vi "ezAFM Practice 1.4.vi"() -> ()   [LabVIEW 2015]
uses:
  D:/LabVIEW for ezAFM/LV-PGC 2019-05a/Special Equipment/ezAFM/NMI Integration Code/ezCommander.dll
  LabVIEW for ezAFM/LV-PGC 2019-05a/Special Equipment/ezAFM/NMI Integration Code/ezCommander.dll
  <vilib>/userdefined/High Color/IMAQdx.ctl
  LabVIEW for ezAFM/LV-PGC 2019-05a/Universal vi's/Global Variables/Globals-EasyAFM.vi
  Globals.vi
  <vilib>/vision/driver/NI_Vision_Acquisition_Software.lvlib
panel:
  in  "Camera":enum32{"ezAFM Camera"}(tab)
  out "ezAFM Camera":T1(plugin-control)
  out "XY Vector":dbl[](array[numeric])
  in  "Main Menu":enum32{"Navigation", "Scanning"}(tab)
  in  "APPROACH":bool
  in  "RETRACT":bool
  in  "Step Size":dbl
  out "Angle":dbl
  in  "THETA":bool
  in  "MOVE":bool
  in  "Current Device":string(combo)
  in  "Target Device":string(combo)
  in  "Motor Speed":u16(ring)=5000 items=["SLOW"=5000, "MEDIUM"=30000, "FAST"=50000]
  in  "Navigation Buttons":T2
  in  "QUIT":bool
  in  "UPDATE DEVICE":bool
  out "Scan Spot":string
  in  "Leads":string(combo)
  in  "Device":string(combo)
  in  "Chip":string
  in  "Image Resolution":u16(ring)=256 items=["32"=32, "64"=64, "128"=128, "256"=256, "512"=512, "1024"=1024, "2048"=2048]
  in  "SELECT CONNECTIONS":bool
  in  "BEGIN SCAN":bool
  out "Current Device to Scan":string
  out "Connections":string[](array[string])
  in  "Indicators":enum32{"Indicators"}(tab)
  out "XYZ Motor Position":dbl[](array[numeric])
  out "ezAFM Status":dbl
  out "Approaching":bool
  out "ezAFM Connected":bool
  out "Retracting":bool
  out "Scanning":bool
  out "Tip Approached?":bool
  in  "RESET":bool
  out "XY Position":dbl[](array[numeric])
  # "Use Arrow Keys to manually\nmove the XY Motor"
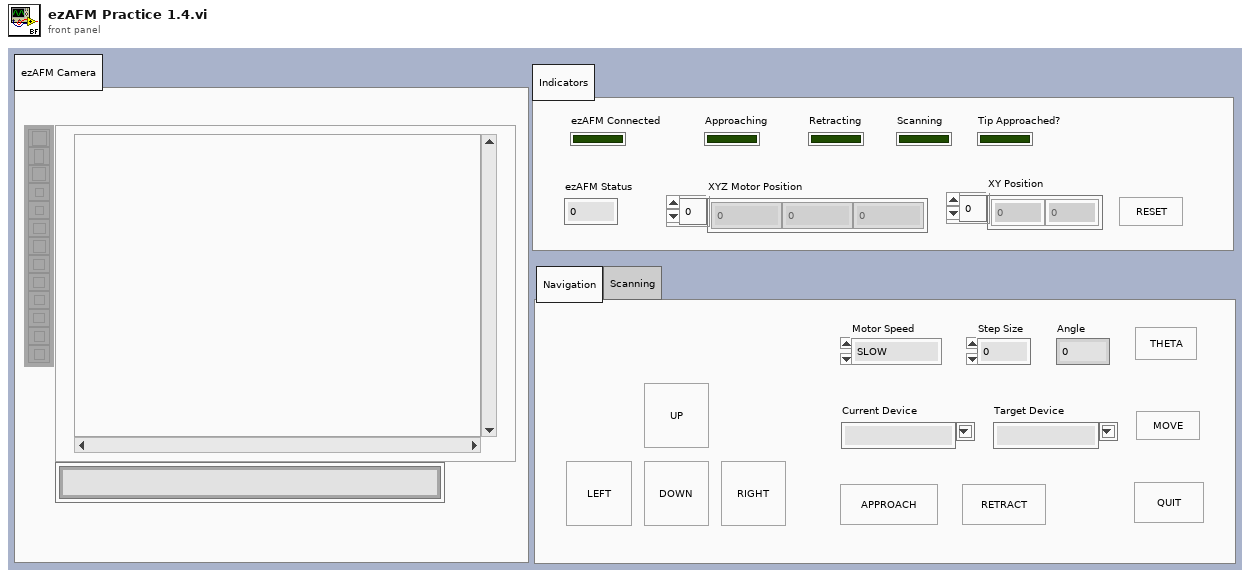
[diagram p1: front panel]
types:
  T1 = typedef "IMAQ Image.ctl" = refnum<image>
  T2 = cluster{"UP":bool, "DOWN":bool, "LEFT":bool, "RIGHT":bool}
  T3 = typedef "IMAQdx.ctl" = refnum<k21>
  T4 = typedef "Image Type" = u32
  T5 = typedef "eventvkey.ctl" = enum16{"ASCII", "Enter", "Return", "Shift", "Ctrl", "Alt", "Cmd", "Opt", "Caps", "NumLock", "Clear", "Break", "Up", "Down", "Left", "Right", "Insert", "Delete", "Home", "End", "PageUp", "PageDown", "Escape", "Help", "Pause", "ScrollLock", "F1", "F2", "F3", "F4", "F5", "F6", "F7", "F8", "F9", "F10", "F11", "F12", "F13", "F14", "F15", "F16", "F17", "F18", "F19", "F20", "F21", "F22", "F23", "F24", "Play", "VolumeUp", "VolumeDown", "Mute", "Two Byte Char"}
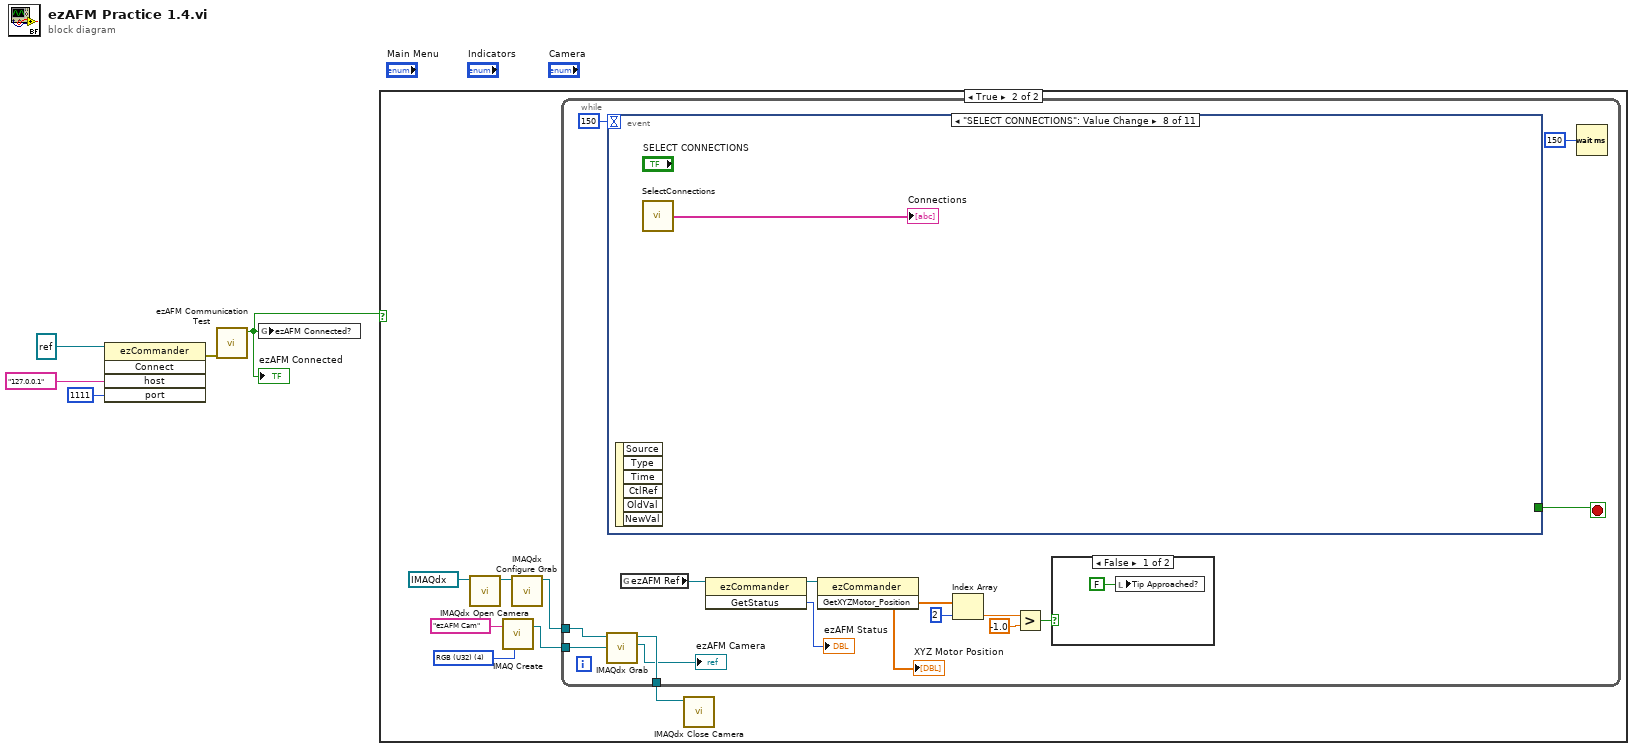
[diagram p0: block diagram]
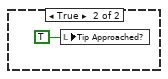
[diagram p3: hidden frame]
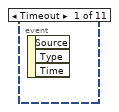
[diagram p4: hidden frame]
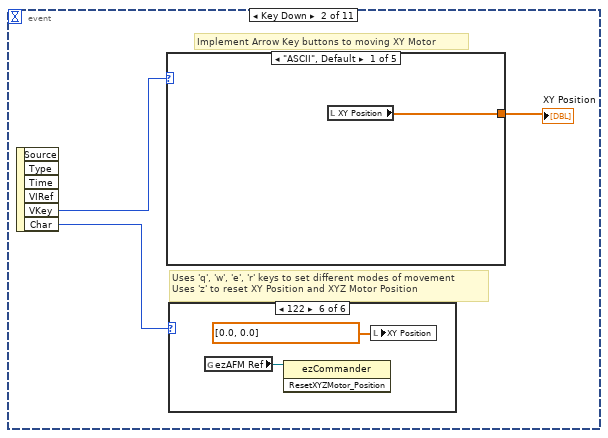
[diagram p5: hidden frame]
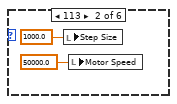
[diagram p7: hidden frame]
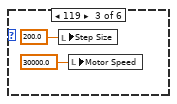
[diagram p8: hidden frame]
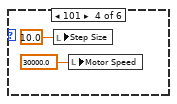
[diagram p9: hidden frame]
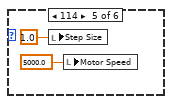
[diagram p10: hidden frame]
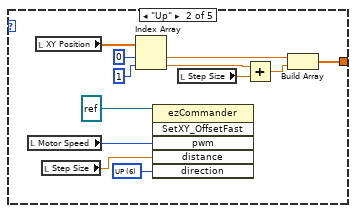
[diagram p11: hidden frame]
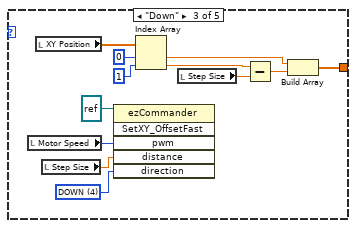
[diagram p12: hidden frame]
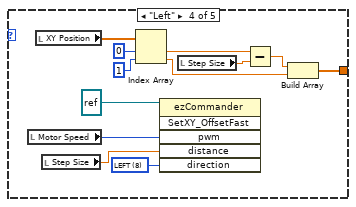
[diagram p13: hidden frame]
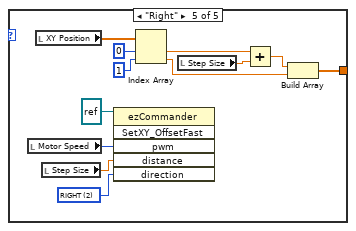
[diagram p14: hidden frame]
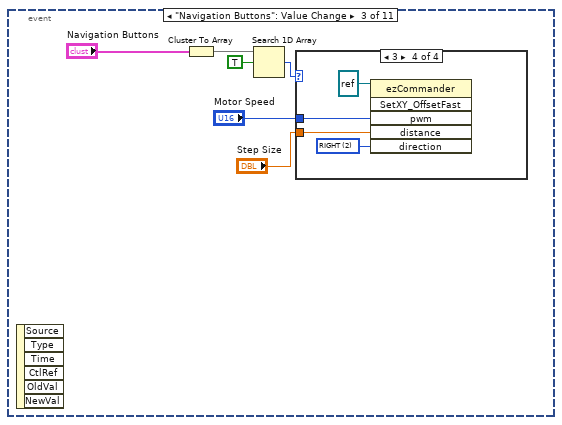
[diagram p15: hidden frame]
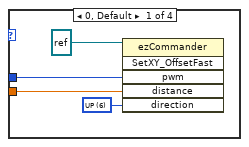
[diagram p16: hidden frame]
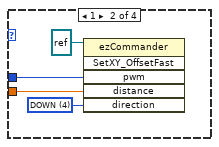
[diagram p17: hidden frame]
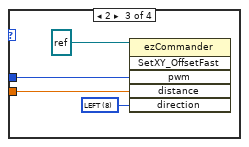
[diagram p18: hidden frame]
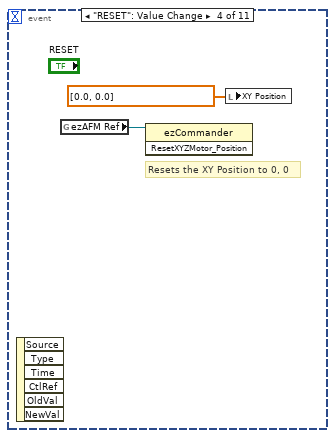
[diagram p19: hidden frame]
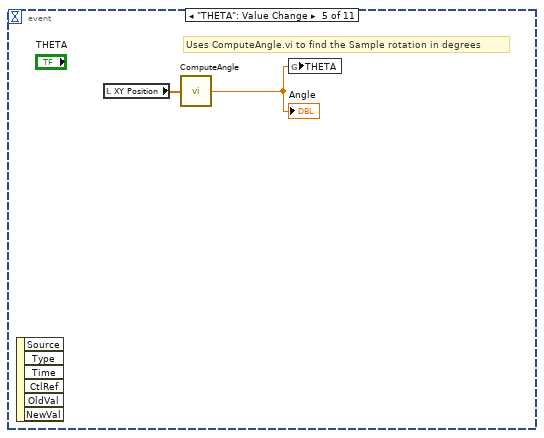
[diagram p20: hidden frame]
diagram:
  n1 = invoke class="ezCommander" method="Connect"(reference=refnum<k24> refnum ("ezAFM Ref"), "host"="127.0.0.1", "port"=1111) -> (error out=w4:errorcluster)  [unwired: 2 in, 4 out]
  n2 = call "ezAFM Communication Test.vi"("error in"=w4) -> ("ezAFM COM status"=w1:bool)  [unwired: 3 in, 3 out]
  "ezAFM Connected" <- w1
  n3 = global write "Globals.vi" "ezAFM Connected?"(w1) -> ()
  n4 = case shown="True" w1 {
    frame False {
    }
    frame True {
      w6 = T4 4 items=["Grayscale (U8)", "Grayscale (I16)", "Grayscale (SGL)", "Complex (CSG)", "RGB (U32)", "HSL (U32)", "RGB (U64)", "Grayscale (U16)"] ("Image Type")
      n5 = call <vilib>:"IMAQdx Open Camera.vi"("Session In"=T3 "cam5") -> ("Session Out"=w10:T3)  [unwired: 9 in, 1 out]
      n6 = call "IMAQ Create"("Image Name"="ezAFM Cam", "Image Type"=w6) -> ("New Image"=w9:T1)  [unwired: 3 in, 1 out]
      n7 = call <vilib>:"IMAQdx Configure Grab.vi"("Session In"=w10) -> ("Session Out"=w8:T3)  [unwired: 9 in, 1 out]
      n8 = while {
        tunnel: w9 -> [w17]
        tunnel: w8 -> [w16]
        tunnel: [w15] -> w7
        stop <- w20 stop-if-true
        n9 = call <vilib>:"IMAQdx Grab.vi"("Image In"=w17, "Session In"=w16) -> ("Image Out"=→"ezAFM Camera":T1, "Session Out"=w15:T3)  [unwired: 2 in, 6 out]
        n10 = event shown="[7] \"SELECT CONNECTIONS\": Value Change" {
          selector: _ -> [_ _ _ _ _ _ _ _ _ _ _]
          dyn-events: _ -> [_ _ _ _ _ _ _ _ _ _ _]
          timeout: 150 -> [_ _ _ _ _ _ _ _ _ _ _]
          tunnel: [_ _ _ _ _ _ _ _ _ _ "QUIT"] -> w20
          event Timeout {
            n11 = event-data() -> ()  [unwired: 1 in, 3 out]
          }
          event Key Down {
            # "Uses 'q', 'w', 'e', 'r' keys to set different modes of movement\nUses 'z' to reset XY Position and XYZ Motor Position"
            # "Implement Arrow Key buttons to moving XY Motor"
            n12 = event-data() -> ("VKey"=w30:T5, "Char"=w31:i16)  [unwired: 1 in, 4 out]
            n13 = case shown="\"ASCII\", Default" w30 {
              tunnel: [w43 w44 w56 w68 w80] -> w32
              frame "ASCII", Default {
                n14 = local read "XY Position"() -> (w43:dbl[])
              }
              frame "Up" {
                w54 = u16 6 items=["UP"=6, "DOWN"=4, "LEFT"=8, "RIGHT"=2]
                n15 = local read "Motor Speed"() -> (w53:u16)
                n16 = local read "XY Position"() -> (w51:dbl[])
                n17 = local read "Step Size"() -> (w52:dbl)
                n18 = Index Array(array=w51, index #1=0 ("index"), index #2=1 ("index")) -> (element #1=w46:dbl, element #2=w47:dbl)
                n19 = invoke class="ezCommander" method="SetXY_OffsetFast"(reference=refnum<k24> refnum ("ezAFM Ref"), "pwm"=w53, "distance"=w52, "direction"=w54) -> ()  [unwired: 2 in, 6 out]
                n20 = local read "Step Size"() -> (w48:dbl)
                n21 = Add(x=w47, y=w48) -> (x+y=w45:dbl)
                n22 = Build Array(w46, w45) -> (w44:dbl[])
              }
              frame "Down" {
                w64 = u16 4 items=["UP"=6, "DOWN"=4, "LEFT"=8, "RIGHT"=2]
                n23 = local read "Motor Speed"() -> (w66:u16)
                n24 = local read "XY Position"() -> (w58:dbl[])
                n25 = local read "Step Size"() -> (w65:dbl)
                n26 = invoke class="ezCommander" method="SetXY_OffsetFast"(reference=refnum<k24> refnum ("ezAFM Ref"), "pwm"=w66, "distance"=w65, "direction"=w64) -> ()  [unwired: 2 in, 6 out]
                n27 = Index Array(array=w58, index #1=0 ("index"), index #2=1 ("index")) -> (element #1=w60:dbl, element #2=w61:dbl)
                n28 = local read "Step Size"() -> (w57:dbl)
                n29 = Subtract(x=w61, y=w57) -> (x-y=w59:dbl)
                n30 = Build Array(w60, w59) -> (w56:dbl[])
              }
              frame "Left" {
                w78 = u16 8 items=["UP"=6, "DOWN"=4, "LEFT"=8, "RIGHT"=2]
                n31 = local read "Motor Speed"() -> (w76:u16)
                n32 = local read "XY Position"() -> (w72:dbl[])
                n33 = local read "Step Size"() -> (w77:dbl)
                n34 = Index Array(array=w72, index #1=0 ("index"), index #2=1 ("index")) -> (element #1=w71:dbl, element #2=w69:dbl)
                n35 = invoke class="ezCommander" method="SetXY_OffsetFast"(reference=refnum<k24> refnum ("ezAFM Ref"), "pwm"=w76, "distance"=w77, "direction"=w78) -> ()  [unwired: 2 in, 6 out]
                n36 = local read "Step Size"() -> (w73:dbl)
                n37 = Subtract(x=w71, y=w73) -> (x-y=w70:dbl)
                n38 = Build Array(w70, w69) -> (w68:dbl[])
              }
              frame "Right" {
                w90 = u16 2 items=["UP"=6, "DOWN"=4, "LEFT"=8, "RIGHT"=2]
                n39 = local read "Motor Speed"() -> (w89:u16)
                n40 = local read "XY Position"() -> (w85:dbl[])
                n41 = local read "Step Size"() -> (w88:dbl)
                n42 = invoke class="ezCommander" method="SetXY_OffsetFast"(reference=refnum<k24> refnum ("ezAFM Ref"), "pwm"=w89, "distance"=w88, "direction"=w90) -> ()  [unwired: 2 in, 6 out]
                n43 = Index Array(array=w85, index #1=0 ("index"), index #2=1 ("index")) -> (element #1=w83:dbl, element #2=w81:dbl)
                n44 = local read "Step Size"() -> (w84:dbl)
                n45 = Add(x=w83, y=w84) -> (x+y=w82:dbl)
                n46 = Build Array(w82, w81) -> (w80:dbl[])
              }
            }
            "XY Position" <- w32
            n47 = case shown="122" w31 {
              frame 0, Default {
              }
              frame 113 {
                n48 = local write "Step Size"(1000.0 ("Step Size")) -> ()
                n49 = local write "Motor Speed"(50000.0 ("Motor Speed")) -> ()
              }
              frame 119 {
                n50 = local write "Step Size"(200.0 ("Step Size")) -> ()
                n51 = local write "Motor Speed"(30000.0 ("Motor Speed")) -> ()
              }
              frame 101 {
                n52 = local write "Step Size"(10.0 ("Step Size")) -> ()
                n53 = local write "Motor Speed"(30000.0 ("Motor Speed")) -> ()
              }
              frame 114 {
                n54 = local write "Step Size"(1.0 ("Step Size")) -> ()
                n55 = local write "Motor Speed"(5000.0 ("Motor Speed")) -> ()
              }
              frame 122 {
                n56 = global read "Globals-EasyAFM.vi" "ezAFM Ref"() -> (w41:refnum<k24>)
                n57 = invoke class="ezCommander" method="ResetXYZMotor_Position"(reference=w41) -> ()  [unwired: 2 in, 3 out]
                n58 = local write "XY Position"(dbl[] [0.0, 0.0] ("XY Position")) -> ()
              }
            }
          }
          event "Navigation Buttons": Value Change {
            n59 = event-data() -> ()  [unwired: 1 in, 6 out]
            n60 = Cluster To Array(cluster="Navigation Buttons") -> (array=w96:bool[])
            n61 = Search 1D Array(1D array=w96, element=TRUE) -> (index of element=w94:i32)  [unwired: 1 in]
            n62 = case shown="3" w94 {
              tunnel: "Step Size" -> [w98 w103 w107 w111]
              tunnel: "Motor Speed" -> [w99 w102 w106 w110]
              frame 0, Default {
                w100 = u16 6 items=["UP"=6, "DOWN"=4, "LEFT"=8, "RIGHT"=2]
                n63 = invoke class="ezCommander" method="SetXY_OffsetFast"(reference=refnum<k24> refnum ("ezAFM Ref"), "pwm"=w99, "distance"=w98, "direction"=w100) -> ()  [unwired: 2 in, 6 out]
              }
              frame 1 {
                w104 = u16 4 items=["UP"=6, "DOWN"=4, "LEFT"=8, "RIGHT"=2]
                n64 = invoke class="ezCommander" method="SetXY_OffsetFast"(reference=refnum<k24> refnum ("ezAFM Ref"), "pwm"=w102, "distance"=w103, "direction"=w104) -> ()  [unwired: 2 in, 6 out]
              }
              frame 2 {
                w108 = u16 8 items=["UP"=6, "DOWN"=4, "LEFT"=8, "RIGHT"=2]
                n65 = invoke class="ezCommander" method="SetXY_OffsetFast"(reference=refnum<k24> refnum ("ezAFM Ref"), "pwm"=w106, "distance"=w107, "direction"=w108) -> ()  [unwired: 2 in, 6 out]
              }
              frame 3 {
                w112 = u16 2 items=["UP"=6, "DOWN"=4, "LEFT"=8, "RIGHT"=2]
                n66 = invoke class="ezCommander" method="SetXY_OffsetFast"(reference=refnum<k24> refnum ("ezAFM Ref"), "pwm"=w110, "distance"=w111, "direction"=w112) -> ()  [unwired: 2 in, 6 out]
              }
            }
          }
          event "RESET": Value Change {
            # "Resets the XY Position to 0, 0"
            n67 = event-data() -> ()  [unwired: 1 in, 6 out]
            n68 = global read "Globals-EasyAFM.vi" "ezAFM Ref"() -> (w114:refnum<k24>)
            n69 = invoke class="ezCommander" method="ResetXYZMotor_Position"(reference=w114) -> ()  [unwired: 2 in, 3 out]
            n70 = local write "XY Position"(dbl[] [0.0, 0.0] ("XY Position")) -> ()
          }
          event "THETA": Value Change {
            # "Uses ComputeAngle.vi to find the Sample rotation in degrees"
            n71 = event-data() -> ()  [unwired: 1 in, 6 out]
            n72 = local read "XY Position"() -> (w117:dbl[])
            n73 = call "ComputeAngle.vi"("XY Vector"=w117) -> ("Angle"=w116:dbl)
            "Angle" <- w116
            n74 = global write "Globals.vi" "THETA"(w116) -> ()
          }
          event "MOVE": Value Change {
            w122 = u16 50000 items=["SLOW"=5000, "MEDIUM"=30000, "FAST"=50000]
            # "XY Vector is in cartesian coordinates of the Oasis Camera\nUses Move2Device.vi to find the XY Vector between the Current Device and Target Device crosshairs\nInputs the XY Vector into Move2Vector.vi to command the XY Motor to move"
            n75 = event-data() -> ()  [unwired: 1 in, 6 out]
            n76 = call "GetDeviceVector.vi"("Target Device"="Target Device", "Current Device"="Current Device") -> ("XY Vector"=w119:dbl[])
            "XY Vector" <- w119
            n77 = local read "Angle"() -> (w118:dbl)
            n78 = call "Move2Vector 2.0.vi"("Angle"=w118, "Motor Speed"=w122, "XY Vector"=w119) -> ()  [unwired: 1 out]
          }
          event "APPROACH", "RETRACT": Value Change {
            n79 = event-data() -> ()  [unwired: 1 in, 6 out]
            n80 = case shown="True" "RETRACT" {
              selector: "RETRACT" -> [_ w125]
              frame False {
              }
              frame True {
                n81 = call "Retract.vi"("Number of Cycles"=10, "Retracting?"=w125) -> ("Finished?"=w127:bool)
                n82 = Not(x=w127) -> (.not. x?=w126:bool)
                n83 = local write "Tip Approached?"(w126) -> ()
                n84 = local write "Retracting"(w126) -> ()
                "Retracting" <- w125
              }
            }
            n85 = case shown="True" "APPROACH" {
              selector: "APPROACH" -> [_ w129]
              frame False {
              }
              frame True {
                n86 = call "AutoLand&Approach.vi"("Approaching?"=w129) -> ("Finished?"=w130:bool)
                "Tip Approached?" <- w130
                n87 = Not(x=w130) -> (.not. x?=w131:bool)
                n88 = local write "Approaching"(w131) -> ()
                "Approaching" <- w129
              }
            }
          }
          event "SELECT CONNECTIONS": Value Change {
            n89 = event-data() -> ()  [unwired: 1 in, 6 out]
            n90 = call "SelectConnections.vi"() -> ("Selected Connections"=→"Connections":string[])  [unwired: 1 in]
          }
          event "UPDATE DEVICE": Value Change {
            n91 = event-data() -> ()  [unwired: 1 in, 6 out]
            n92 = local read "Device"() -> (w134:string)
            n93 = local read "Leads"() -> (w133:string)
            n94 = Concatenate Strings("Chip", w134, w133) -> (→"Current Device to Scan":string)
            n95 = case shown="\"abcde\"" "Leads" {
              tunnel: ["None" "A" ("string") "B" ("string")] -> w135
              frame "None", Default {
              }
              frame "abcde" {
              }
              frame "efgh" {
              }
            }
            n96 = String Length(string="Device") -> (length=w138:i32)
            n97 = Decrement(x=w138) -> (x-1=w137:i32)
            n98 = String Subset(string="Device", offset (0)=w137) -> (substring=w136:string)  [unwired: 1 in]
            n99 = case shown="\"1\", \"3\"" w136 {
              tunnel: w135 -> [w144 w146 w149]
              tunnel: [w144 w145 w148] -> w141
              frame "None", Default {
              }
              frame "0", "2" {
                n100 = Concatenate Strings(w146, "1" ("string")) -> (w145:string)
              }
              frame "1", "3" {
                n101 = Concatenate Strings(w149, "2" ("string")) -> (w148:string)
              }
            }
            "Scan Spot" <- w141
          }
          event "BEGIN SCAN": Value Change {
            n102 = event-data() -> ("NewVal"=→"Scanning":bool)  [unwired: 1 in, 5 out]
            n103 = flat-sequence {
              frame #0 {
                w157 = u16 5000 items=["SLOW"=5000, "MEDIUM"=30000, "FAST"=50000]
                # "Scan Region 1"
                # "Move to the target spot"
                n104 = local read "Scan Spot"() -> (w158:string)
                n105 = case shown="\"None\", Default" w158 {
                  tunnel: [dbl[] [0.0, 0.0] dbl[] [-73.0, 35.0] dbl[] [-73.0, -56.0] dbl[] [-55.0, 35.0] dbl[] [-55.0, -56.0]] -> w155
                  frame "None", Default {
                  }
                  frame "A1" {
                  }
                  frame "A2" {
                  }
                  frame "B1" {
                  }
                  frame "B2" {
                  }
                }
                n106 = local read "Angle"() -> (w156:dbl)
                n107 = call "Move2Vector 2.0.vi"("Angle"=w156, "Motor Speed"=w157, "XY Vector"=w155) -> ()  [unwired: 1 out]
                n108 = local write "XY Vector"(w155) -> ()
              }
              frame #1 {
                n109 = local read "Current Device to Scan"() -> (w165:string)
                n110 = local read "Angle"() -> (w167:dbl)
                n111 = call "Scan3Regions.vi"("Angle"=w167, "Image Resolution"="Image Resolution", "Current Device to Scan"=w165) -> ("Finished?"=w164:bool)
                n112 = local write "Scanning"(w164) -> ()
              }
            }
          }
          event "QUIT": Value Change {
            w168 = FALSE ("ezAFM Connected?")
            n113 = event-data() -> ()  [unwired: 1 in, 6 out]
            n114 = global write "Globals.vi" "ezAFM Connected?"(w168) -> ()
            n115 = local write "ezAFM Connected"(w168) -> ()
          }
        }
        n116 = global read "Globals-EasyAFM.vi" "ezAFM Ref"() -> (w22:refnum<k24>)
        n117 = invoke class="ezCommander" method="GetStatus"(reference=w22) -> (reference out=w21:refnum<k24>, "GetStatus"=→"ezAFM Status":i32)  [unwired: 2 in, 1 out]
        n118 = invoke class="ezCommander" method="GetXYZMotor_Position"(reference=w21) -> ("GetXYZMotor_Position"=w23:dbl[])  [unwired: 2 in, 2 out]
        "XYZ Motor Position" <- w23
        n119 = Index Array(array=w23, index=2) -> (element=w24:dbl)
        n120 = Greater?(x=w24, y=-1.0) -> (0:w25:bool)
        n121 = case shown="False" w25 {
          frame False {
            n122 = local write "Tip Approached?"(FALSE ("Tip Approached?")) -> ()
          }
          frame True {
            n123 = local write "Tip Approached?"(TRUE ("Tip Approached?")) -> ()
          }
        }
        n124 = Wait (ms)(milliseconds to wait=u32 150) -> ()  [unwired: 1 out]
      }
      n125 = call <vilib>:"IMAQdx Close Camera.vi"("Session In"=w7) -> ()  [unwired: 10 in, 1 out]
    }
  }
